vi "MedianFilter.vi"(0 "Numeric 9":dbl, 1 "vHL":sgl, 5 "Numeric 7":dbl, 7 "Numeric 5":dbl, 9 "Numeric 3":dbl, 11 "Numeric in":dbl) -> (4 "Numeric 10":dbl, 6 "Numeric 8":dbl, 8 "Numeric 6":dbl, 10 "Numeric 4":dbl, 14 "OUTPUT":dbl, 15 "Numeric 2":dbl)   [LabVIEW 2016]
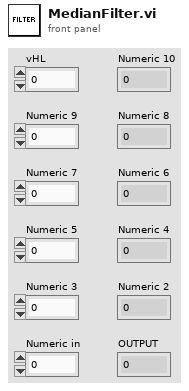
[diagram p1: front panel]
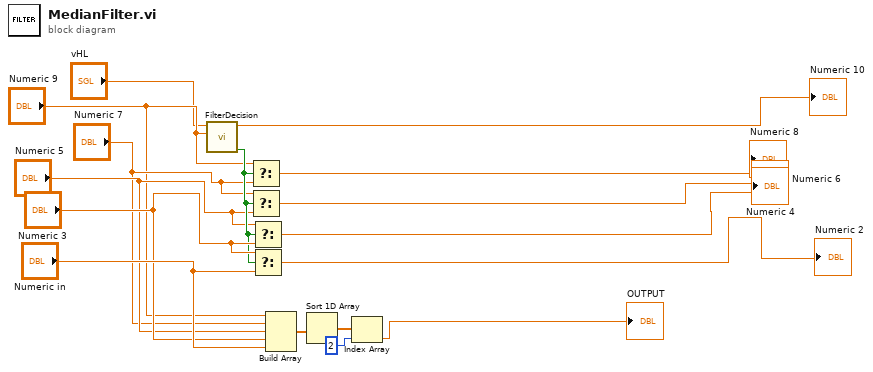
[diagram p0: block diagram]
diagram:
  n1 = call "FilterDecision.vi"("vHL in"="Numeric 9", "vHL 3"="vHL") -> ("Boolean"=w12:bool, "vHL out"=→"Numeric 10":dbl)  [unwired: 8 in]
  n2 = Select(t="Numeric 9", s=w12, f="Numeric 7") -> (s? t:f=→"Numeric 8":dbl)
  n3 = Select(t="Numeric 7", s=w12, f="Numeric 5") -> (s? t:f=→"Numeric 6":dbl)
  n4 = Select(t="Numeric 5", s=w12, f="Numeric 3") -> (s? t:f=→"Numeric 4":dbl)
  n5 = Select(t="Numeric 3", s=w12, f="Numeric in") -> (s? t:f=→"Numeric 2":dbl)
  n6 = Build Array("Numeric 9", "Numeric 7", "Numeric 5", "Numeric 3", "Numeric in") -> (w5:dbl[])
  n7 = Sort 1D Array(array=w5) -> (sorted array=w1:dbl[])
  n8 = Index Array(array=w1, index=2) -> (element=→"OUTPUT":dbl)
